vi "get_all_calib.vi"(0 "VISA resource name":refnum<visa-resource-name>, 1 "error in (no error)":errorcluster) -> (2 "VISA resource Salida":refnum<visa-resource-name>, 3 "Gains":dbl[](array[numeric]), 4 "Offsets":dbl[](array[numeric]), 5 "error out":errorcluster)   [LabVIEW 2011]
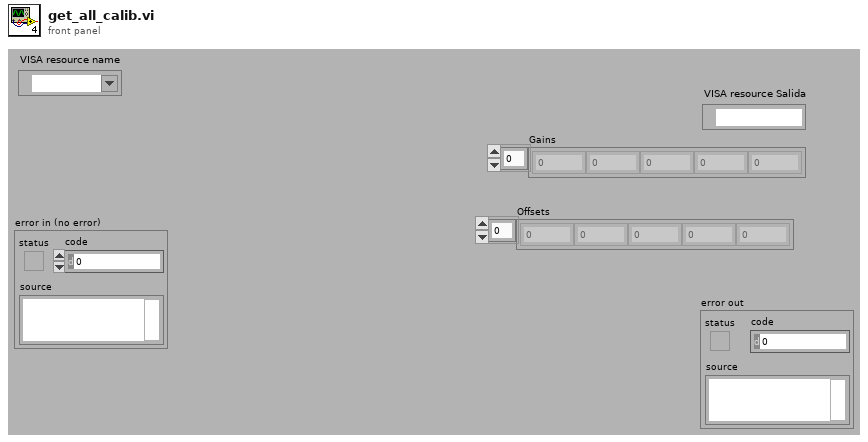
[diagram p1: front panel]
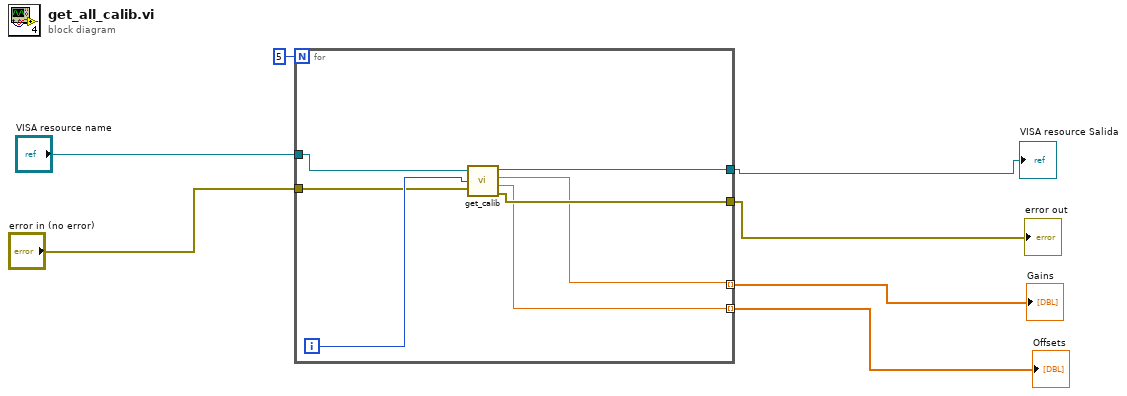
[diagram p0: block diagram]
diagram:
  n1 = for {
    N: 5 -> [_]
    tunnel: "VISA resource name" -> [w12]
    tunnel: "error in (no error)" -> [w13]
    tunnel: [w11] -> w4
    tunnel: [w10] -> w3
    tunnel: [w9] -> w1 mode=indexing
    tunnel: [w8] -> w2 mode=indexing
    i -> [w14]
    n2 = call "get_calib.vi"("VISA resource name"=w12, "Gain"=w14, "error in (no error)"=w13) -> ("VISA resource Salida"=w11:refnum<visa-resource-name>, "slope"=w8:dbl, "offset"=w9:dbl, "error out"=w10:errorcluster)
  }
  "error out" <- w3
  "VISA resource Salida" <- w4
  "Gains" <- w2
  "Offsets" <- w1
